vi "Delete.vi"(0 "video writer in":refnum<class "MSC Video Writer.lvclass">, 5 "error in (no error)":errorcluster) -> (19 "error out":errorcluster)   [LabVIEW 2014, in "MSC Video Writer.lvclass"]
doc: "Ends the Video Writer Operation and deletes the reference to it.\nUse this function for each initialized video writer to prevent memory leaks.\nDoes not delete the saved file."
uses:
  MSC Video Writer.lvclass
  MSC Video Writer.lvclass/MSC Video Writer.ctl
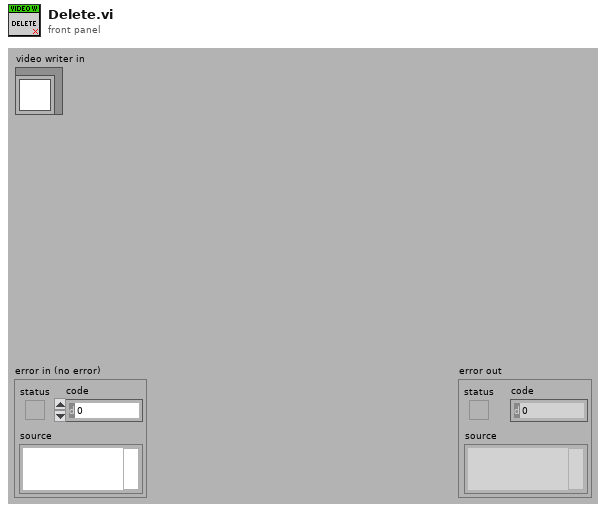
[diagram p1: front panel]
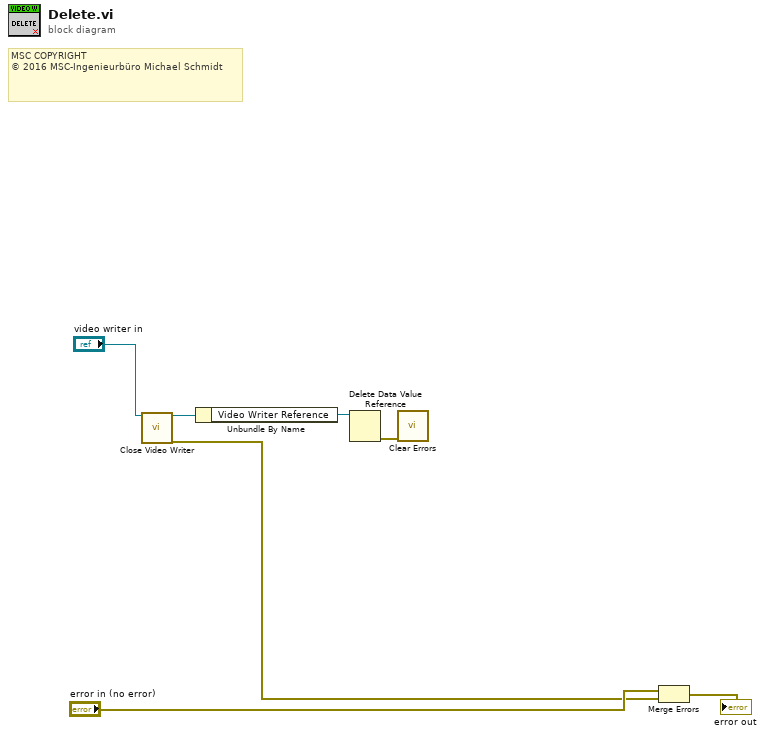
[diagram p0: block diagram]
diagram:
  # "MSC COPYRIGHT\n© 2016 MSC-Ingenieurbüro Michael Schmidt"
  # "MSC COPYRIGHT\n© 2016 MSC-Ingenieurbüro Michael Schmidt"
  n1 = call "Close Video Writer.vi"("video writer in"="video writer in") -> ("video writer out"=w1:refnum<class "MSC Video Writer.lvclass">, "error out"=w3:errorcluster)  [unwired: 17 in]
  n2 = Unbundle By Name(w1) -> ("Video Writer Reference"=w4:refnum<data-value>)
  n3 = Delete Data Value Reference(data value reference=w4) -> (error out=w5:errorcluster)  [unwired: 1 in, 1 out]
  n4 = call <vilib>:"Clear Errors.vi"("error in (no error)"=w5) -> ()  [unwired: 5 in, 2 out]
  n5 = Merge Errors("error in (no error)", w3) -> (→"error out":errorcluster)
